vi "risingEdgeCounter32Bit.vi"(2 "In":bool, 3 "Reset":bool) -> (0 "32BitCounter":u32)   [LabVIEW 2014]
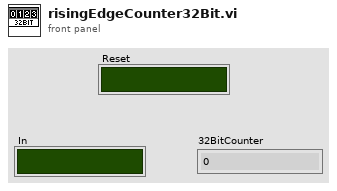
[diagram p1: front panel]
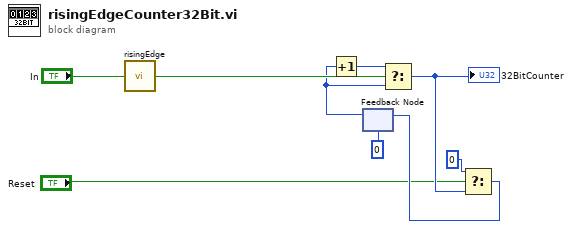
[diagram p0: block diagram]
diagram:
  n1 = call "risingEdge.vi"("In"="In") -> ("out"=w8:bool)
  n2 = feedback #1(u32 0) -> (w7:u32)
  n3 = Increment(x=w7) -> (x+1=w6:u32)
  n4 = Select(t=w6, s=w8, f=w7) -> (s? t:f=w4:u32)
  "32BitCounter" <- w4
  n5 = Select(t=u32 0, s="Reset", f=w4) -> (s? t:f=w5:u32)
  n6 = feedback-in #1(w5) -> ()
